vi "CreateNewLayer.vi"(6 "Insert Position (0)":i32, 8 "error in":errorcluster, 9 "Force New Layer?":bool, 11 "Icon.lvclass":refnum<class "Icon.lvclass">) -> (0 "error out":errorcluster, 1 "#Layers":i32, 3 "Icon.lvclass out":refnum<class "Icon.lvclass">, 4 "Layer added?":bool)   [LabVIEW 2021, in "Icon.lvclass"]
doc: "Create a new User Layer"
uses:
  <vilib>/LabVIEW Icon API/lv_icon/Classes/Icon/Icon.lvclass
  <vilib>/LabVIEW Icon API/lv_icon/Controls/LayerType.ctl
  <vilib>/LabVIEW Icon API/lv_icon/Classes/Layer/Layer.lvclass
  <vilib>/LabVIEW Icon API/lv_icon/lv_icon.lvlib
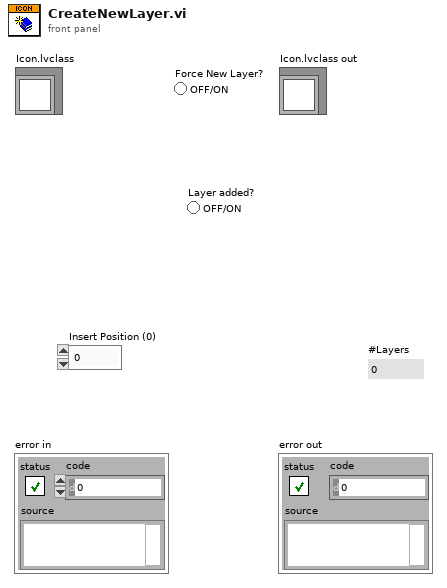
[diagram p1: front panel]
types:
  T1 = typedef "LayerType.ctl" = enum16{"Graphic", "Text", "Tool", "Graphic Drop"}
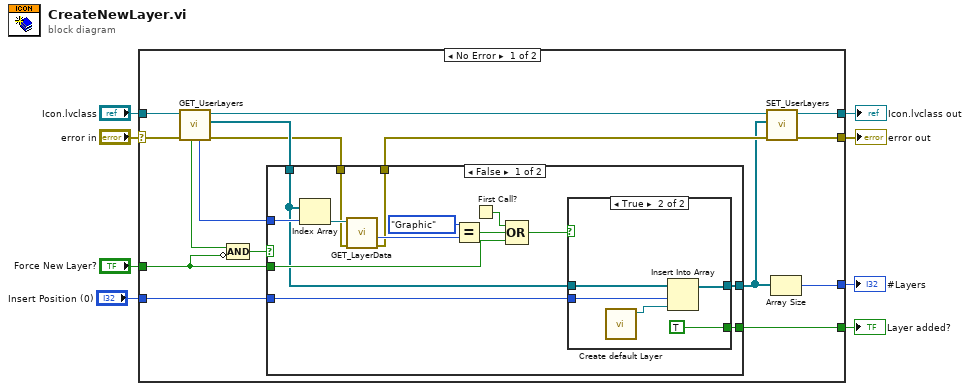
[diagram p0: block diagram]
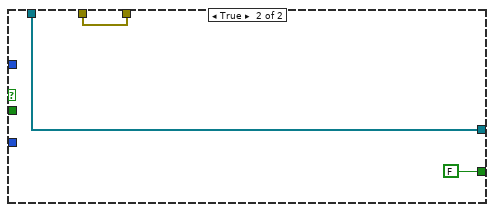
[diagram p3: hidden frame]
diagram:
  n1 = case shown="No Error" "error in" {
    selector: "error in" -> [w21 w48]
    tunnel: [w24 w49] -> w8
    tunnel: "Icon.lvclass" -> [w20 w49]
    tunnel: [w23 w48] -> w6
    tunnel: "Force New Layer?" -> [w9 _]
    tunnel: [w17 _] -> w3
    tunnel: "Insert Position (0)" -> [w14 _]
    tunnel: [w12 _] -> w1
    frame No Error {
      n2 = call-dynamic "GET_UserLayers.vi"("error in (no error)"=w21, "Icon.lvclass in"=w20) -> ("error out"=w16:errorcluster, "All Layers"=w18:refnum<class "Layer.lvclass">[], "Icon.lvclass out"=w22:refnum<class "Icon.lvclass">, "#Active Layer"=w19:i32, "Layer Locked?"=w11:bool)  [unwired: 5 out]
      n3 = Compound Arithmetic op=AND(w11, invert w9) -> (w10:bool)
      n4 = case shown="False" w10 {
        tunnel: w9 -> [w38 _]
        tunnel: w19 -> [w37 _]
        tunnel: w18 -> [w31 w46]
        tunnel: [w30 FALSE] -> w17
        tunnel: w16 -> [w29 w47]
        tunnel: [w28 w47] -> w15
        tunnel: w14 -> [w27 _]
        tunnel: [w26 w46] -> w13
        frame False {
          n5 = Index Array(array=w31, index=w37) -> (element=w36:refnum<class "Layer.lvclass">)
          n6 = call-dynamic "GET_LayerData.vi"("error in (no error)"=w29, "Layer.lvclass in"=w36) -> ("error out"=w28:errorcluster, "Type"=w35:T1)  [unwired: 8 out]
          n7 = Equal?(x=LayerType."Graphic" ("y"), y=w35) -> (x = y?=w33:bool)
          n8 = First Call?() -> (First Call?: T/F=w32:bool)
          n9 = Compound Arithmetic op=OR(w32, w33, w38) -> (w25:bool)
          n10 = case shown="True" w25 {
            tunnel: [w39 w40] -> w26
            tunnel: w31 -> [w39 w43]
            tunnel: [_ TRUE] -> w30
            tunnel: w27 -> [_ w42]
            frame False {
            }
            frame True {
              n11 = call <vilib>:"Create default Layer.vi"() -> ("Layer.lvclass out"=w41:refnum<class "Layer.lvclass">)  [unwired: 1 in, 10 out]
              n12 = Insert Into Array(array=w43, index=w42, new element=w41) -> (w40:refnum<class "Layer.lvclass">[])
            }
          }
        }
        frame True {
        }
      }
      n13 = call-dynamic "SET_UserLayers.vi"("error in (no error)"=w15, "Layers"=w13, "Icon.lvclass in"=w22) -> ("error out"=w23:errorcluster, "Icon.lvclass out"=w24:refnum<class "Icon.lvclass">)  [unwired: 1 in, 6 out]
      n14 = Array Size(array=w13) -> (size(s)=w12:i32)
    }
    frame Error {
    }
  }
  "Icon.lvclass out" <- w8
  "error out" <- w6
  "Layer added?" <- w3
  "#Layers" <- w1
